vi "Stop Core.vi"(10 "final error code":i32, 11 "Test_Caller in":refnum<class "Test_Caller.lvclass">) -> (3 "Test_Caller out":refnum<class "Test_Caller.lvclass">)   [LabVIEW 2025, in "Test_Caller.lvlib" / "Test_Caller.lvclass"]
doc: "<p>(<strong>Filename</strong>: <span class=\"dnl\">Actor Framework.lvlib:Actor.lvclass:Stop Core.vi</span>)</p>\n<p>Defines what the actor does before it stops. Use the <strong>final error code</strong> input to determine whether the actor shut down in response to an error.</p>\n<p>By default, this method passes the Stop message along to all <a href=\"nihelplauncher://docs/csh?context=lvcore_lvcomm_af_launch_nested_actor\">auto-stop nested actors</a>. A descendant class may override this method to define additional behavior, such as shutting down any processes the actor initiated in its override of the <a href=\"nihelplauncher://docs/csh?context=lvcore_lvcomm_af_actor_core\">Actor Core</a> method.</p>"
uses:
  Test_Caller.lvclass
  Test_Caller.lvclass/Test_Caller.ctl
  <vilib>/ActorFramework/Actor/Actor.lvclass
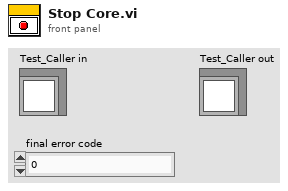
[diagram p1: front panel]
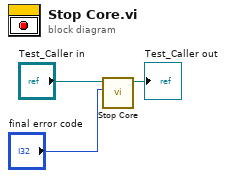
[diagram p0: block diagram]
diagram:
  n1 = call-parent "Stop Core.vi"("final error code"="final error code", "Actor in"="Test_Caller in") -> ("Actor out"=→"Test_Caller out":refnum<class "Test_Caller.lvclass">)  [unwired: 9 in]
